vi "Idle_Data_Read_Setup (SubVI).vi"(0 "Sampling Time":dbl=1.0, 5 "Temperature Freq":dbl=30.0, 7 "Pressure Freq":dbl=30.0, 11 "error in (no error)":errorcluster) -> (1 "Pressure Task 2":refnum<k21>, 2 "task out":refnum<k21>, 3 "Samples Per Channel":dbl, 4 "Refnum out":refnum<k21>, 6 "Pressure Task":refnum<k21>, 8 "Pressure Samples":dbl, 10 "Temperature Task":refnum<k21>, 12 "Temperature Samples":dbl, 13 "error out":errorcluster, 14 "error out 2":errorcluster, 15 "error out":errorcluster)   [LabVIEW 2018]
uses:
  <vilib>/DAQmx/create/channels.llb/DAQmx Create Channel (AI-Voltage-Basic).vi
  <vilib>/DAQmx/configure/timing.llb/DAQmx Timing (Sample Clock).vi
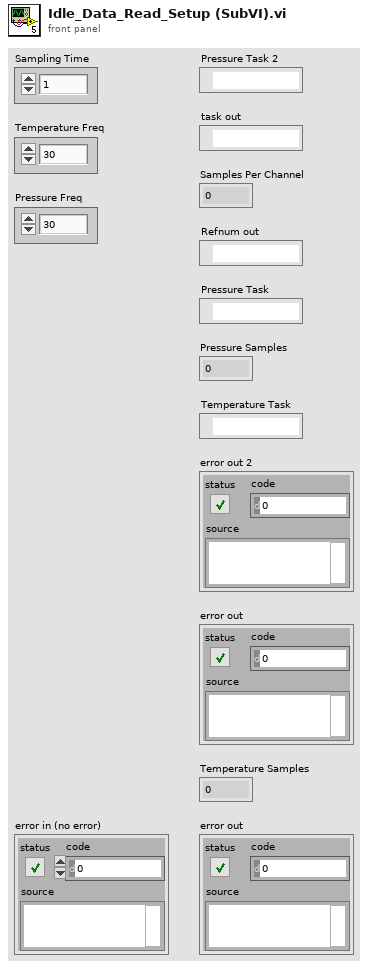
[diagram p1: front panel]
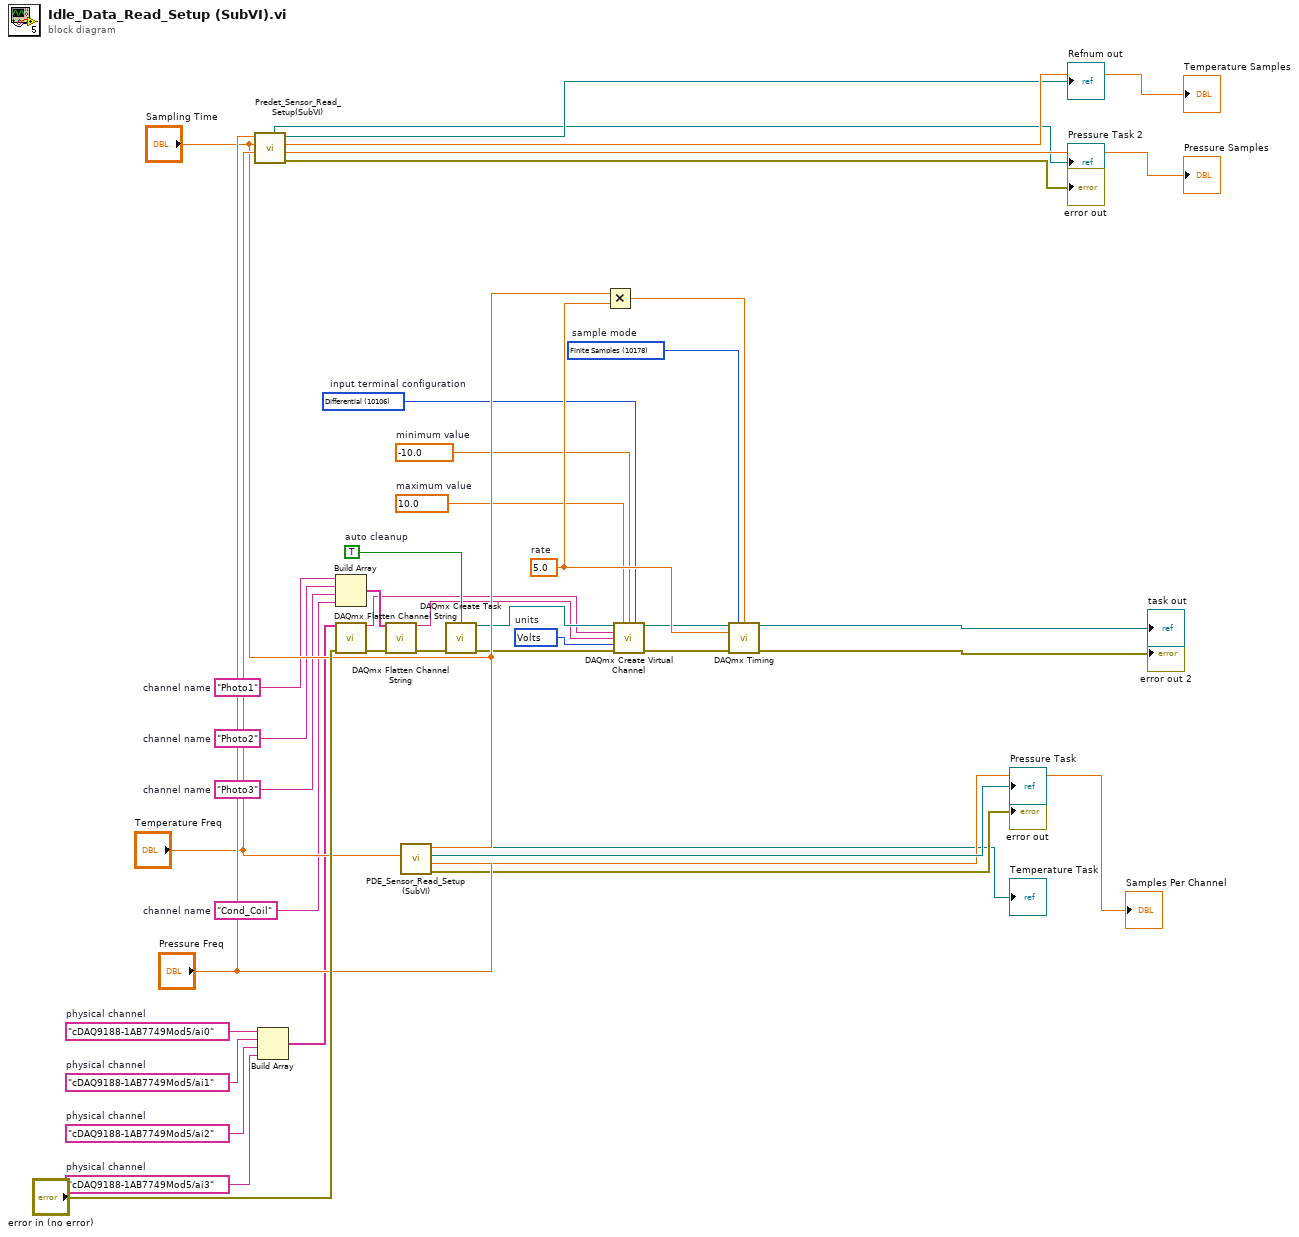
[diagram p0: block diagram]
diagram:
  w30 = 10178 items=["Finite Samples"=10178, "Continuous Samples"=10123, "Hardware Timed Single Point"=12522]  # sample mode
  w27 = 5.0  # rate
  w18 = "Cond_Coil"  # channel name
  w10 = "cDAQ9188-1AB7749Mod5/ai3"  # physical channel
  w19 = "Photo3"  # channel name
  w13 = "cDAQ9188-1AB7749Mod5/ai2"  # physical channel
  w20 = "Photo2"  # channel name
  w14 = "cDAQ9188-1AB7749Mod5/ai1"  # physical channel
  w25 = 10106 items=["default"=-1, "RSE"=10083, "NRSE"=10078, "Differential"=10106, "Pseudodifferential"=12529]  # input terminal configuration
  w22 = 10348 items=["Volts"=10348, "From Custom Scale"=10065]  # units
  w21 = "Photo1"  # channel name
  w24 = -10.0  # minimum value
  w23 = 10.0  # maximum value
  w12 = "cDAQ9188-1AB7749Mod5/ai0"  # physical channel
  w32 = TRUE  # auto cleanup
  n1 = call "Predet_Sensor_Read_Setup(SubVI).vi"("Temperature Freq"="Temperature Freq", "Sampling Time"="Sampling Time", "Pressure Freq"="Pressure Freq") -> ("error out"=→"error out":errorcluster, "Pressure Samples"=→"Pressure Samples":dbl, "Temperature Samples"=→"Temperature Samples":dbl, "Temperature Task"=→"Refnum out":refnum<k21>, "Pressure Task"=→"Pressure Task 2":refnum<k21>)  [unwired: 4 in]
  n2 = Build Array(w12, w14, w13, w10) -> (w15:string[])
  n3 = Build Array(w21, w20, w19, w18) -> (w17:string[])
  n4 = call <vilib>:"DAQmx Flatten Channel String.vi"("names in"=w15, "error in"="error in (no error)") -> ("names out"=w11:string, "error out"=w6:errorcluster)  [unwired: 12 in]
  n5 = call <vilib>:"DAQmx Flatten Channel String.vi"("names in"=w17, "error in"=w6) -> ("names out"=w16:string, "error out"=w7:errorcluster)  [unwired: 12 in]
  n6 = call "PDE_Sensor_Read_Setup (SubVI).vi"("Pressure Freq"="Pressure Freq", "Temperature Freq"="Temperature Freq", "Sampling Time"="Sampling Time") -> ("error out"=→"error out":errorcluster, "Samples Per Channel"=→"Samples Per Channel":dbl, "Pressure Task"=→"Pressure Task":refnum<k21>, "Temperature Task"=→"Temperature Task":refnum<k21>)  [unwired: 5 in]
  n7 = call <vilib>:"DAQmx Create Task.vi"("auto cleanup"=w32, "error in"=w7) -> ("task out"=w31:refnum<k21>, "error out"=w33:errorcluster)  [unwired: 12 in]
  n8 = Multiply(x="Sampling Time", y=w27) -> (x*y=w26:dbl)
  n9 = call-poly <vilib>:"DAQmx Create Virtual Channel.vi"("task in"=w31, "maximum value"=w23, "minimum value"=w24, "input terminal configuration"=w25, "physical channels"=w11, "name to assign"=w16, "units"=w22, "error in"=w33) -> ("task out"=w9:refnum<k21>, "error out"=w8:errorcluster)  [unwired: 6 in]
  n10 = call-poly <vilib>:"DAQmx Timing.vi"("task/channels in"=w9, "sample mode"=w30, "samples per channel"=w26, "rate"=w27, "error in"=w8) -> ("task out"=→"task out":refnum<k21>, "error out"=→"error out 2":errorcluster)  [unwired: 9 in]
